vi "Script Editor Dialog.vi"(5 "VI Refnum":refnum<vi>, 7 "Name(\"\" to use uuid)":string="script_editor", 8 "Error in":errorcluster caption="Error in (no error)", 11 "Script":string="Data: Initialize\nInitialize Core Data\nEvents: Register\nUI: Initialize\nUI: Front Panel State >> Open") -> (0 "Error out":errorcluster, 3 "Script out":string)   [LabVIEW 2017]
uses:
  _Support/Priority Queue/Priority Queue.lvclass/Priority Queue.ctl
  AdvanceAPI/CSM - Keywords.vi
  _Support/Common/Trim Single line Text.vi
  AdvanceAPI/CSM - Check If Module Exists.vi
  Utility/Build Error Cluster.vi
  _Support/Process/CSMP-Sync Call.vi
  Utility/uuid.vi
  Utility/Trim Both Whitespace.vi
  _Support/CSMQ/_Obtain CSM Data Queue.vi
  _Support/Priority Queue/Release Priority Queue.vi
  _Support/CSMQ/_CSMObj-Message Check.vi
  _Support/CSMQ/_CSMObj-Enqueue Cross-Module Message.vi
  _Support/CSMQ/_CSMOFGV Get.vi
  _Support/Priority Queue/Obtain Priority Queue.vi
  _Support/Priority Queue/Enqueue Element.vi
  AdvanceAPI/CSM - Replace Substitution Marks in Messages.vi
  _Support/CSMQ/_CSMOFGV.vi
  _Support/Error/CSM No Target Error.vi
  _Support/Error/CSM Not Allowed Message.vi
  _Support/Message/global-TMO for Sync-Rep.vi
  _Support/Priority Queue/Priority Queue.lvclass
  Communicable State Machine.lvlib
panel:
  in  "Script List":i32(listbox)
  in  "Delete 3":bool
  in  "Delete 2":bool
  in  "Add Back":bool
  in  "Delete":bool
  in  "Add Front":bool
  in  "Replace":bool
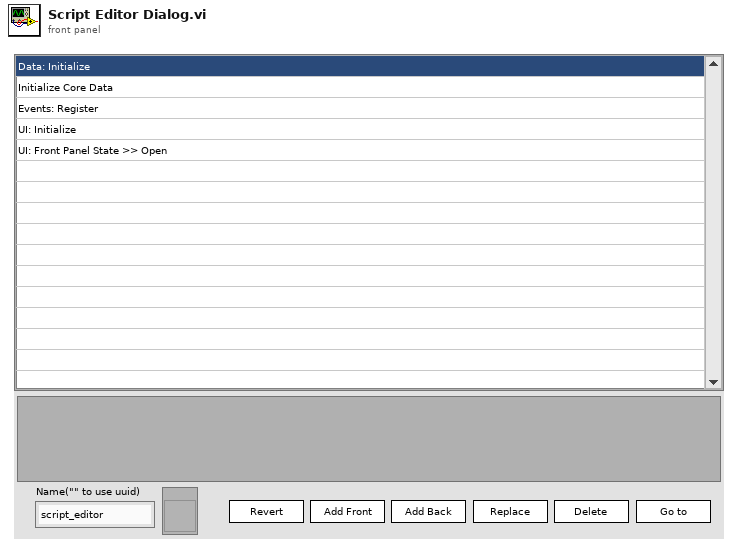
[diagram p1: front panel]
types:
  T1 = enum32{"Invalid", "Standard", "Closed", "Hidden", "Minimized", "Maximized"}
  T2 = enum32{"invalid app kind", "Development System", "Run Time System", "Student Edition", "Embedded LabVIEW", "Evaluation", "Custom"}
  T3 = typedef "Communicable State Machine.lvlib/_CSM_Response Source Message.ctl" = cluster{"‘State":string, "’Arguments":string, "’Error":errorcluster}
  T4 = cluster{"Current VI Reference":refnum<vi>, "Close Panel on Exit?":bool}
  T5 = cluster{"Core":cluster{"Current VI Reference":refnum<vi>, "Close Panel on Exit?":bool}, "Script":string}
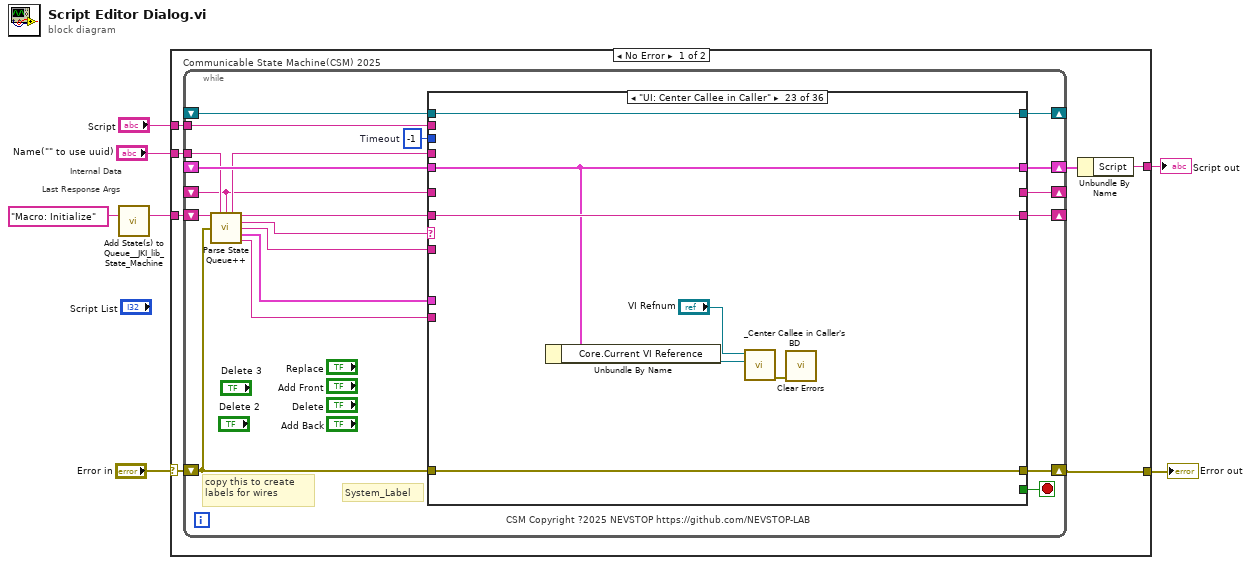
[diagram p0: block diagram]
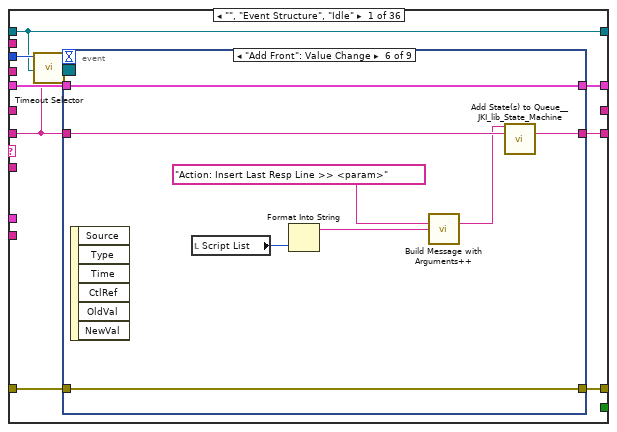
[diagram p2: hidden frame]
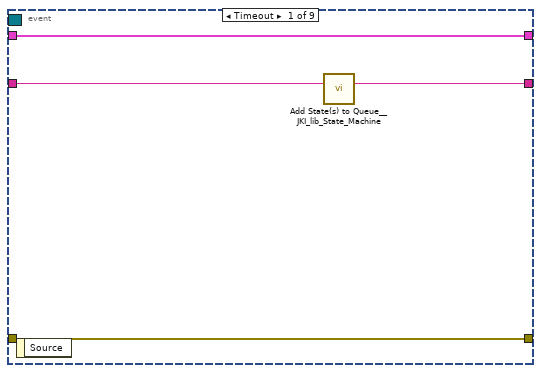
[diagram p3: hidden frame]
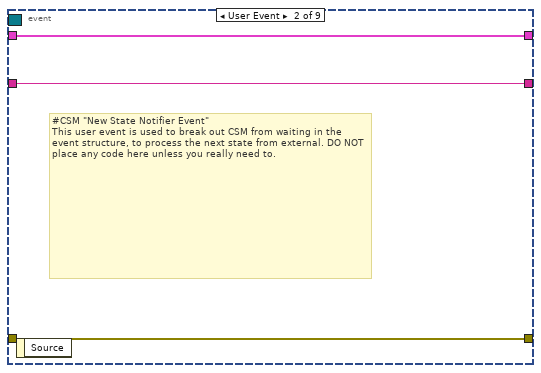
[diagram p4: hidden frame]
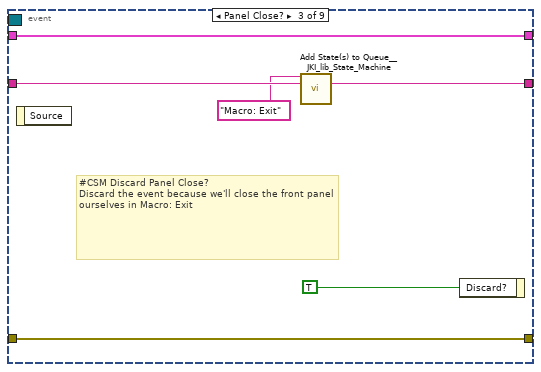
[diagram p5: hidden frame]
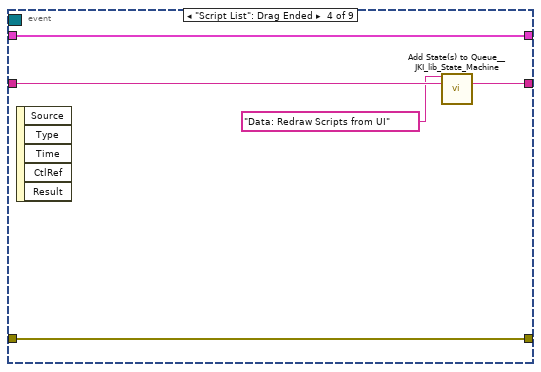
[diagram p6: hidden frame]
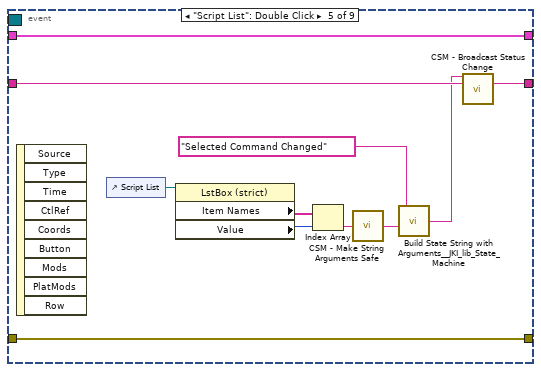
[diagram p7: hidden frame]
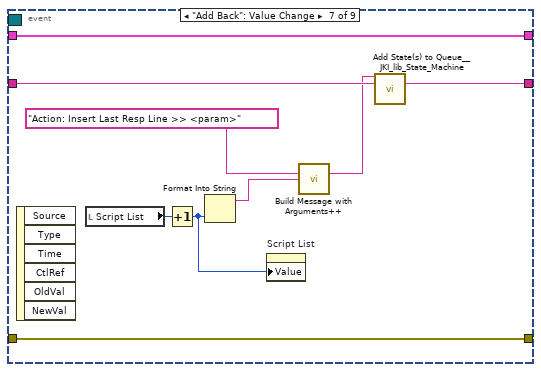
[diagram p8: hidden frame]
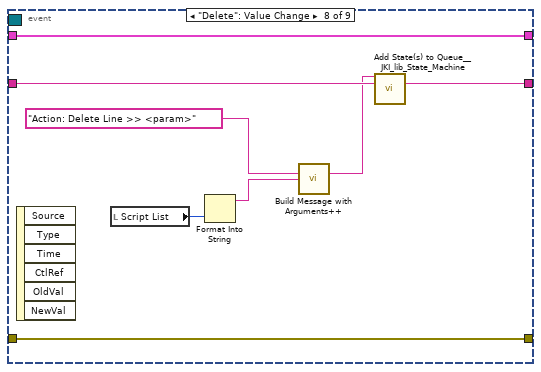
[diagram p9: hidden frame]
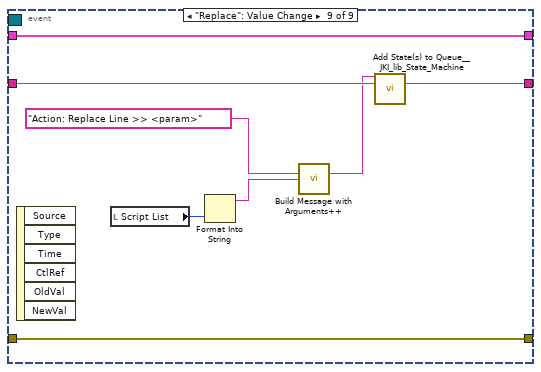
[diagram p10: hidden frame]
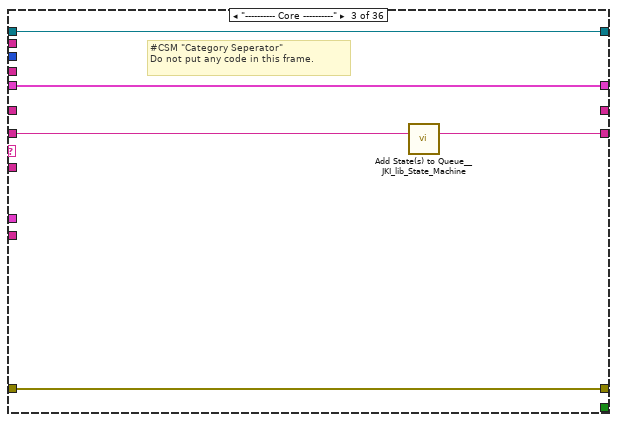
[diagram p12: hidden frame]
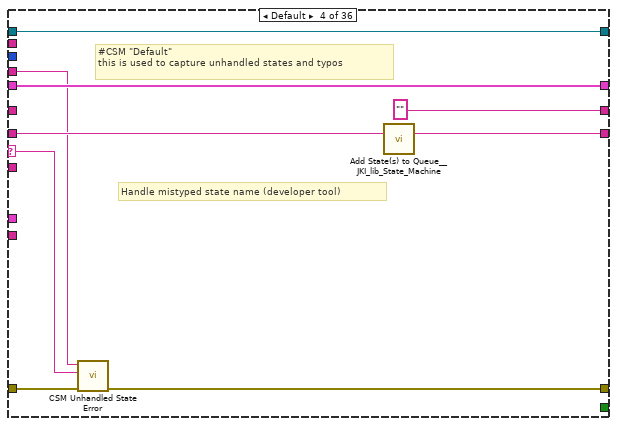
[diagram p13: hidden frame]
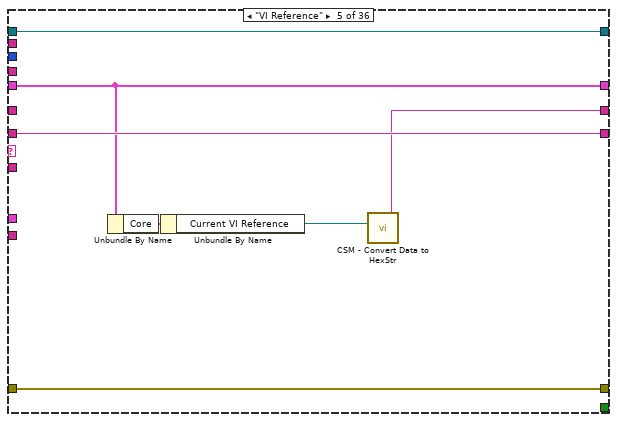
[diagram p14: hidden frame]
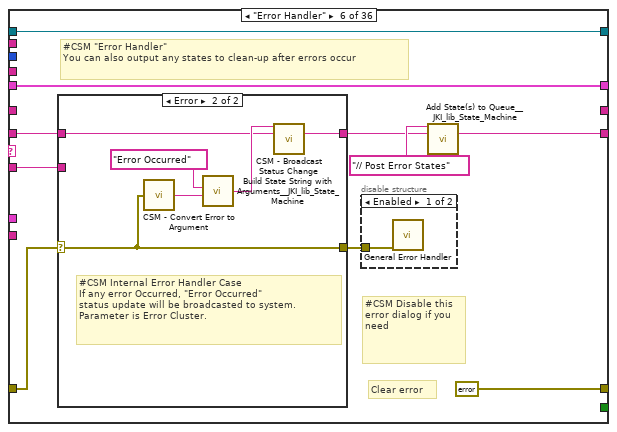
[diagram p15: hidden frame]
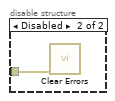
[diagram p16: hidden frame]
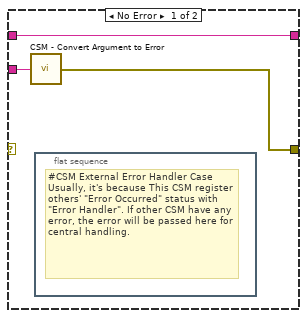
[diagram p17: hidden frame]
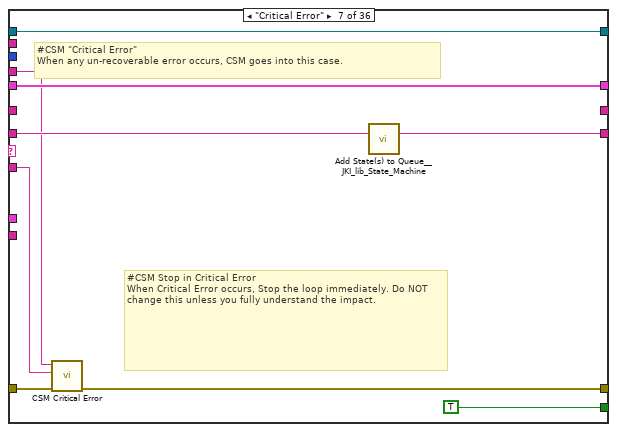
[diagram p18: hidden frame]
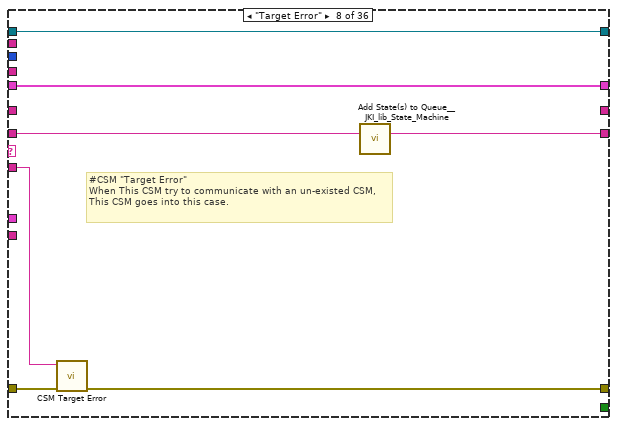
[diagram p19: hidden frame]
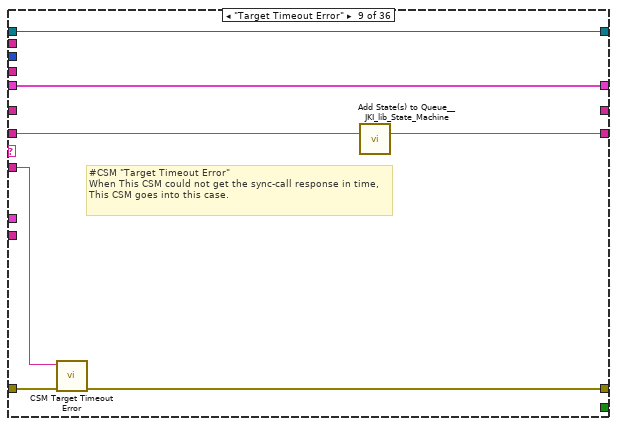
[diagram p20: hidden frame]
diagram:
  # "Last Response Args"
  # "Internal Data"
  n1 = call <vilib>:"Add State(s) to Queue__JKI_lib_State_Machine.vi"("State(s) in (\"\")"="Macro: Initialize" ("Init State(\"Macro: Initialize\")")) -> ("States Out"=w7:string)  [unwired: 14 in]
  n2 = case shown="No Error" "Error in" {
    selector: "Error in" -> [w11 w489]
    tunnel: w7 -> [w14 _]
    tunnel: "Name(\"\" to use uuid)" -> [w13 _]
    tunnel: [w12 w489] -> w4
    tunnel: [w9 w488] -> w2
    tunnel: "Script" -> [w8 w488]
    frame No Error {
      n3 = while "Communicable State Machine(CSM) 2025" {
        shift-right: [w29] -> w10
        shift-left: _ -> [w28]
        shift-right: [w32] -> w12
        shift-left: w11 -> [w26]
        shift-right: [w31] -> _
        shift-left: w14 -> [w33]
        tunnel: w13 -> [w22]
        shift-right: [w25] -> _
        shift-left: _ -> [w16]
        shift-right: [w24] -> _
        shift-left: _ -> [w23]
        tunnel: w8 -> [w15]
        stop <- w30 stop-if-true
        w27 = -1  # Timeout
        # "copy this to create labels for wires"
        # "System_Label"
        # "CSM Copyright ?2025 NEVSTOP https://github.com/NEVSTOP-LAB"
        n4 = call "Parse State Queue++.vi"("State Queue"=w33, "Name(\"\" to use uuid)"=w22, "Response Arguments"=w16, "Previous Error"=w26) -> ("Name Used"=w17:string, "Remaining States"=w34:string, "Current State"=w21:string, "Arguments"=w20:string, ">> Response Source Message >>"=w19:T3, ">> Source CSM >>"=w18:string)  [unwired: 6 in]
        n5 = case shown="\"UI: Center Callee in Caller\"" w21 {
          selector: w21 -> [_ _ _ w117 _ _ _ _ _ _ _ _ _ _ _ _ _ _ _ _ _ _ _ _ _ _ _ _ _ _ _ _ _ _ _ _]
          tunnel: w34 -> [w35 w108 w114 w122 w129 w135 w158 w164 w171 w180 w193 w208 w214 w219 w226 w233 w241 w246 w253 w257 w263 w270 w276 w279 w291 w307 w379 w401 w407 w421 w424 w427 w439 w457 w475 w487]
          tunnel: w20 -> [_ _ _ _ _ w134 w153 w163 w170 w179 _ _ _ _ _ _ _ _ _ _ _ _ _ _ w286 w301 _ _ _ _ _ w429 _ w453 w470 w482]
          tunnel: w28 -> [w42 w107 w111 w120 w128 w139 w159 w166 w173 w182 w192 w201 w212 w216 _ w232 w236 w243 w252 w256 w260 w266 w274 w283 w289 w303 w396 w398 w404 w418 w423 w433 w436 w455 w472 w484]
          tunnel: [w41 w109 w112 w115 w130 errorcluster {"status"=FALSE, "code"=0, "source"=""} ("error out") w154 w161 w168 w185 w194 w205 w211 w217 w223 w234 w237 w244 w247 w255 w261 w268 w277 w284 w287 w304 w378 w399 w405 w419 w425 w434 w437 w444 w473 w485] -> w32
          tunnel: w26 -> [w40 w109 w112 w123 w130 w136 w160 w162 w169 _ w194 w205 w211 w217 w223 w234 w238 w244 _ w258 w261 w268 w277 w284 w288 w305 _ w399 w405 w419 w425 w434 w437 _ w473 w485]
          tunnel: [w43 w108 w113 w121 w129 w131 w157 w167 w174 w181 w193 w207 w213 w218 w225 w233 w240 w245 w253 w257 w262 w269 w276 w280 w290 w306 w380 w400 w406 w420 w424 w428 w438 w456 w474 w486] -> w31
          tunnel: [_ _ _ _ _ _ TRUE _ _ _ _ _ TRUE _ _ _ _ _ _ _ _ _ _ _ _ _ _ _ _ _ _ _ _ _ _ _] -> w30
          tunnel: [w39 w107 w111 w120 w128 w139 w159 w166 w173 w183 w192 w206 w212 w216 w224 w228 w236 w243 w252 w256 w260 w266 w274 w283 w289 w303 w396 w398 w404 w418 w423 w431 w436 w455 w472 w484] -> w29
          tunnel: w27 -> [w38 _ _ _ _ _ _ _ _ _ _ _ _ _ _ _ _ _ _ _ _ _ _ _ _ _ _ _ _ _ _ _ _ _ _ _]
          tunnel: w18 -> [_ _ _ _ _ _ _ _ _ w177 _ _ _ _ _ _ _ _ _ _ _ _ _ _ _ _ _ _ _ _ _ _ _ _ _ _]
          tunnel: w19 -> [_ _ _ _ _ _ _ _ _ w184 _ _ _ _ _ _ _ _ _ _ _ _ _ _ _ _ _ _ _ _ _ _ _ _ _ _]
          tunnel: [_ _ _ "" w124 _ _ _ _ _ _ _ _ _ _ _ _ _ _ _ _ _ _ _ _ _ _ _ _ _ _ _ _ _ _ _] -> w25
          tunnel: [w37 w106 w110 w118 w127 w138 w155 w165 w172 w186 w191 w195 w209 w215 w221 w231 w235 w242 w251 w254 w259 w267 w275 w282 w285 w300 w395 w397 w402 w411 w422 w432 w435 w454 w471 w483] -> w24
          tunnel: w23 -> [w37 w106 w110 w118 w127 w138 w155 w165 w172 w186 w191 w195 w209 w215 w221 w231 w235 w242 _ w254 w259 w267 w275 w282 w285 w300 w395 w397 w402 w411 w422 w432 w435 w454 w471 w483]
          tunnel: w17 -> [_ _ _ w116 _ _ w152 _ _ _ _ _ _ _ _ _ _ _ w250 _ _ _ _ _ _ _ w384 _ _ w410 _ _ _ w443 w461 _]
          tunnel: w16 -> [_ _ _ _ _ _ _ _ _ _ _ _ _ _ _ _ _ _ _ _ _ _ _ _ _ _ _ _ _ _ _ _ _ _ _ _]
          tunnel: w15 -> [_ _ _ _ _ _ _ _ _ _ _ _ _ _ w220 _ _ _ _ _ _ _ _ _ _ _ _ _ _ _ _ _ _ _ _ _]
          frame "", "Event Structure", "Idle" {
            n6 = call "Timeout Selector.vi"("Remaining States"=w35, "Timeout Expected"=w38) -> ("Timeout"=w36:i32)  [unwired: 5 in]
            n7 = event shown="[5] \"Add Front\": Value Change" {
              selector: w37 -> [_ _ _ _ _ _ _ _ _]
              dyn-events: _ -> [_ _ _ _ _ _ _ _ _]
              timeout: w36 -> [_ _ _ _ _ _ _ _ _]
              tunnel: w35 -> [w47 w49 w56 w58 w69 w77 w86 w94 w102]
              tunnel: [w46 w49 w55 w59 w70 w78 w87 w95 w103] -> w43
              tunnel: w42 -> [w44 w50 w53 w60 w71 w79 w88 w96 w104]
              tunnel: [w45 w48 w54 w61 w72 w80 w89 w97 w105] -> w41
              tunnel: w40 -> [w45 w48 w54 w61 w72 w80 w89 w97 w105]
              tunnel: [w44 w50 w53 w60 w71 w79 w88 w96 w104] -> w39
              event Timeout {
                n8 = event-data() -> ()  [unwired: 1 in, 1 out]
                n9 = call <vilib>:"Add State(s) to Queue__JKI_lib_State_Machine.vi"("State(s) in (\"\")"=w47) -> ("States Out"=w46:string)  [unwired: 14 in]
              }
              event User Event {
                # "#CSM \"New State Notifier Event\"\nThis user event is used to break out CSM from waiting in the event structure, to process the next state from external. DO NOT place any code here unless you really need to."
                n10 = event-data() -> ()  [unwired: 1 in, 1 out]
              }
              event Panel Close? {
                # "#CSM Discard Panel Close?\nDiscard the event because we'll close the front panel ourselves in Macro: Exit"
                n11 = event-data() -> ()  [unwired: 1 in, 1 out]
                n12 = call <vilib>:"Add State(s) to Queue__JKI_lib_State_Machine.vi"("State(s) in Front (\"\")"="Macro: Exit", "State(s) in (\"\")"=w56) -> ("States Out"=w55:string)  [unwired: 13 in]
                n13 = event-data("Discard?"=TRUE) -> ()  [unwired: 1 in, 1 out]
              }
              event "Script List": Drag Ended {
                n14 = event-data() -> ()  [unwired: 1 in, 5 out]
                n15 = call <vilib>:"Add State(s) to Queue__JKI_lib_State_Machine.vi"("State(s) in Front (\"\")"="Data: Redraw Scripts from UI" ("State(s) in Front (\"\")"), "State(s) in (\"\")"=w58) -> ("States Out"=w59:string)  [unwired: 13 in]
              }
              event "Script List": Double Click {
                n16 = event-data() -> ()  [unwired: 1 in, 9 out]
                n17 = control-ref of="Script List"() -> (w65:refnum<vi>)
                n18 = property class="LstBox (strict)"(reference=w65) -> ("Item Names"=w68:string[], "Value"=w67:i32)  [unwired: 1 in, 2 out]
                n19 = Index Array(array=w68, index=w67) -> (element=w66:string)
                n20 = call "CSM - Make String Arguments Safe.vi"("Argurment String"=w66) -> ("Safe Argurment String"=w64:string)  [unwired: 8 in]
                n21 = call <vilib>:"Build State String with Arguments__JKI_lib_State_Machine.vi"("Arguments (\"\")"=w64, "State"="Selected Command Changed") -> ("State with Arguments"=w62:string)  [unwired: 4 in]
                n22 = call "CSM - Broadcast Status Change.vi"("Status with Arguments"=w62, "State Queue"=w69) -> ("Remaining States"=w70:string)  [unwired: 13 in]
              }
              event "Add Front": Value Change {
                n23 = event-data() -> ()  [unwired: 1 in, 6 out]
                n24 = local read "Script List"() -> (w74:i32)
                n25 = Format Into String(w74) -> (resulting string=w73:string)  [unwired: 3 in, 1 out]
                n26 = call-poly "Build Message with Arguments++.vi"("States with Replace Token"="Action: Insert Last Resp Line >> <param>" ("State(s) in Front (\"\")"), "<param>"=w73) -> ("States"=w75:string)  [unwired: 13 in]
                n27 = call <vilib>:"Add State(s) to Queue__JKI_lib_State_Machine.vi"("State(s) in Front (\"\")"=w75, "State(s) in (\"\")"=w77) -> ("States Out"=w78:string)  [unwired: 13 in]
              }
              event "Add Back": Value Change {
                n28 = event-data() -> ()  [unwired: 1 in, 6 out]
                n29 = local read "Script List"() -> (w83:i32)
                n30 = Increment(x=w83) -> (x+1=w81:i32)
                n31 = Format Into String(w81) -> (resulting string=w82:string)  [unwired: 3 in, 1 out]
                n32 = property on="Script List" class="LstBox (strict)"("Value"=w81) -> ()  [unwired: 2 in, 2 out]
                n33 = call-poly "Build Message with Arguments++.vi"("States with Replace Token"="Action: Insert Last Resp Line >> <param>" ("State(s) in Front (\"\")"), "<param>"=w82) -> ("States"=w84:string)  [unwired: 13 in]
                n34 = call <vilib>:"Add State(s) to Queue__JKI_lib_State_Machine.vi"("State(s) in Front (\"\")"=w84, "State(s) in (\"\")"=w86) -> ("States Out"=w87:string)  [unwired: 13 in]
              }
              event "Delete": Value Change {
                n35 = event-data() -> ()  [unwired: 1 in, 6 out]
                n36 = local read "Script List"() -> (w91:i32)
                n37 = Format Into String(w91) -> (resulting string=w90:string)  [unwired: 3 in, 1 out]
                n38 = call-poly "Build Message with Arguments++.vi"("States with Replace Token"="Action: Delete Line >> <param>" ("State(s) in Front (\"\")"), "<param>"=w90) -> ("States"=w92:string)  [unwired: 13 in]
                n39 = call <vilib>:"Add State(s) to Queue__JKI_lib_State_Machine.vi"("State(s) in Front (\"\")"=w92, "State(s) in (\"\")"=w94) -> ("States Out"=w95:string)  [unwired: 13 in]
              }
              event "Replace": Value Change {
                n40 = event-data() -> ()  [unwired: 1 in, 6 out]
                n41 = local read "Script List"() -> (w99:i32)
                n42 = Format Into String(w99) -> (resulting string=w98:string)  [unwired: 3 in, 1 out]
                n43 = call-poly "Build Message with Arguments++.vi"("States with Replace Token"="Action: Replace Line >> <param>" ("State(s) in Front (\"\")"), "<param>"=w98) -> ("States"=w100:string)  [unwired: 13 in]
                n44 = call <vilib>:"Add State(s) to Queue__JKI_lib_State_Machine.vi"("State(s) in Front (\"\")"=w100, "State(s) in (\"\")"=w102) -> ("States Out"=w103:string)  [unwired: 13 in]
              }
            }
          }
          frame "CSM Documentation" {
            # "#CSM README FIRST\n\nCommunicable State Machine(CSM) is a LabVIEW application framework that builds upon JKI State Machine(JKISM). It follows the pattern of JKISM and extends the keywords to describe message communication between modules, including concepts such as Sync-Message, Async-Message, Subscription/Unsubscription of status - essential elements for creating reusable code modules. For more information, please visit the CSM wiki: https://nevstop-lab.github.io/CSM-Wiki/\n\nFor instructions on JKI State Machine, visit: http://jki.net/state-machine/\nFor information about CSM, visit: https://github.com/NEVSTOP-LAB"
            # "#CSM \"Documentation\"\nCase for holding CSM Documenation"
          }
          frame "---------- Core ----------" {
            # "#CSM \"Category Seperator\"\nDo not put any code in this frame."
            n45 = call <vilib>:"Add State(s) to Queue__JKI_lib_State_Machine.vi"("State(s) in (\"\")"=w114) -> ("States Out"=w113:string)  [unwired: 14 in]
          }
          frame Default {
            # "#CSM \"Default\"\nthis is used to capture unhandled states and typos"
            # "Handle mistyped state name (developer tool)"
            n46 = call "CSM Unhandled State Error.vi"("error in (no error)"=w123, "Current State"=w117, "CSM Name"=w116) -> ("error out"=w115:errorcluster)  [unwired: 8 in]
            n47 = call <vilib>:"Add State(s) to Queue__JKI_lib_State_Machine.vi"("State(s) in (\"\")"=w122) -> ("States Out"=w121:string)  [unwired: 14 in]
          }
          frame "VI Reference" {
            n48 = Unbundle By Name(w128) -> ("Core"=w126:T4)
            n49 = Unbundle By Name(w126) -> ("Current VI Reference"=w125:refnum<vi>)
            n50 = call "CSM - Convert Data to HexStr.vi"("Variant"=w125) -> ("HEX String (0-9,A-F)"=w124:string)  [unwired: 8 in]
          }
          frame "Error Handler" {
            # "#CSM Disable this error dialog if you need"
            # "#CSM \"Error Handler\"\nYou can also output any states to clean-up after errors occur"
            # "Clear error"
            n51 = case shown="Error" w136 {
              selector: w136 -> [_ w146]
              tunnel: [w145 w148] -> w132
              tunnel: w135 -> [w145 w147]
              tunnel: w134 -> [w144 _]
              tunnel: [w143 w146] -> w137
              frame No Error {
                n52 = call "CSM - Convert Argument to Error.vi"("Argument"=w144) -> ("error"=w143:errorcluster)  [unwired: 4 in]
                n53 = flat-sequence {
                  frame #0 {
                    # "#CSM External Error Handler Case\nUsually, it's because This CSM register others' \"Error Occurred\" status with \"Error Handler\". If other CSM have any error, the error will be passed here for central handling."
                  }
                }
              }
              frame Error {
                # "#CSM Internal Error Handler Case \nIf any error Occurred, \"Error Occurred\" \nstatus update will be broadcasted to system.\nParameter is Error Cluster."
                n54 = call "CSM - Convert Error to Argument.vi"("error"=w146) -> ("Argument"=w150:string)  [unwired: 4 in]
                n55 = call <vilib>:"Build State String with Arguments__JKI_lib_State_Machine.vi"("Arguments (\"\")"=w150, "State"="Error Occurred" ("Status with Arguments")) -> ("State with Arguments"=w149:string)  [unwired: 4 in]
                n56 = call "CSM - Broadcast Status Change.vi"("Status with Arguments"=w149, "State Queue"=w147) -> ("Remaining States"=w148:string)  [unwired: 13 in]
              }
            }
            n57 = disable-structure shown="Enabled" {
              disable-tunnel: w137 -> [w141 w142]
              frame Enabled {
                n58 = call <vilib>:"General Error Handler.vi"("error in (no error)"=w141) -> ()  [unwired: 10 in, 5 out]
              }
              frame Disabled {
                n59 = call <vilib>:"Clear Errors.vi"("error in (no error)"=w142) -> ()  [unwired: 5 in, 2 out]
              }
            }
            n60 = call <vilib>:"Add State(s) to Queue__JKI_lib_State_Machine.vi"("State(s) in Front (\"\")"="// Post Error States", "State(s) in (\"\")"=w132) -> ("States Out"=w131:string)  [unwired: 13 in]
          }
          frame "Critical Error" {
            # "#CSM Stop in Critical Error\nWhen Critical Error occurs, Stop the loop immediately. Do NOT change this unless you fully understand the impact."
            # "#CSM \"Critical Error\"\nWhen any un-recoverable error occurs, CSM goes into this case."
            n61 = call "CSM Critical Error.vi"("error in (no error)"=w160, "Arugments(as Reason)"=w153, "CSM Name"=w152) -> ("error out"=w154:errorcluster)  [unwired: 8 in]
            n62 = call <vilib>:"Add State(s) to Queue__JKI_lib_State_Machine.vi"("State(s) in (\"\")"=w158) -> ("States Out"=w157:string)  [unwired: 14 in]
          }
          frame "Target Error" {
            # "#CSM \"Target Error\"\nWhen This CSM try to communicate with an un-existed CSM, This CSM goes into this case."
            n63 = call "CSM Target Error.vi"("error in (no error)"=w162, "Arguments(as CSM Name)"=w163) -> ("error out"=w161:errorcluster)  [unwired: 9 in]
            n64 = call <vilib>:"Add State(s) to Queue__JKI_lib_State_Machine.vi"("State(s) in (\"\")"=w164) -> ("States Out"=w167:string)  [unwired: 14 in]
          }
          frame "Target Timeout Error" {
            # "#CSM \"Target Timeout Error\"\nWhen This CSM could not get the sync-call response in time, This CSM goes into this case."
            n65 = call "CSM Target Timeout Error.vi"("error in (no error)"=w169, "Arguments(as CSM Name)"=w170) -> ("error out"=w168:errorcluster)  [unwired: 9 in]
            n66 = call <vilib>:"Add State(s) to Queue__JKI_lib_State_Machine.vi"("State(s) in (\"\")"=w171) -> ("States Out"=w174:string)  [unwired: 14 in]
          }
          frame "Async Response", "Response" {
            n67 = Unbundle(w184) -> ("‘State"=w178:string, "’Arguments"=w176:string, "’Error"=w175:errorcluster)
            n68 = case shown="Default" w178 {
              tunnel: [w190] -> w185
              tunnel: w175 -> [w190]
              tunnel: [w189] -> w183
              tunnel: w182 -> [w189]
              tunnel: [w187] -> w181
              tunnel: w180 -> [w188]
              tunnel: w179 -> [_]
              tunnel: w177 -> [_]
              tunnel: w176 -> [_]
              frame Default {
                # "#CSM Response Comments\nAfter Message is executed, CSM goes to this state for receive the response.\n    For Async Message(->), \"Async Response\" is used. This CSM will goes to \"Async Message Posted\" immediately and receive the \"Async Response\" after the callee finishes the message.\n    For Sync Message(@),  This CSM will wait until the message is done and immediately goes to \"Response\""
                # "#CSM \"Async Response\"\nHandle Async-call Response (\"Async Response\" for ->)"
                # "#CSM \"Response\"\nHandle Sync-call Response (\"Response\" for -@)"
                n69 = call <vilib>:"Add State(s) to Queue__JKI_lib_State_Machine.vi"("State(s) in (\"\")"=w188) -> ("States Out"=w187:string)  [unwired: 14 in]
              }
            }
          }
          frame "Async Message Posted" {
            # "#CSM \"Async Message Posted\"\nAfter Async Message is posted (-> or ->| ), CSM goes to this state for post-action.\nYou can use Argument - State to tell which Async Message is called."
          }
          frame "Initialize Core Data" {
            # "#CSM \"Initialize Core Data\"\nThis is used to determine panel behavior on exit"
            # "originally closed?"
            # "exe?"
            # "If panel starts closed or is an EXE, then close it when we exit"
            n70 = property class="VI"() -> ("FP.State"=w198:T1)  [unwired: 2 in, 2 out]
            n71 = property class="App"() -> ("App.Kind"=w204:T2)  [unwired: 2 in, 2 out]
            n72 = control-ref of="Current VI Reference"() -> (w199:refnum<vi>)
            n73 = Equal?(x=w198, y=T1."Closed" ("Front Panel Window:State")) -> (x = y?=w196:bool)
            n74 = Equal?(x=w204, y=T2."Run Time System" ("Application:Kind")) -> (x = y?=w202:bool)
            n75 = Or(x=w196, y=w202) -> (x .or. y?=w200:bool)
            n76 = Bundle By Name(cluster=w201, "Core.Current VI Reference"=w199, "Core.Close Panel on Exit?"=w200) -> (w206:T5)
            n77 = call <vilib>:"Add State(s) to Queue__JKI_lib_State_Machine.vi"("State(s) in (\"\")"=w208) -> ("States Out"=w207:string)  [unwired: 14 in]
          }
          frame "Exit" {
            # "#CSM \"Exit\"\nCase for exiting the loop. No errors that occur here will be handled."
            n78 = call <vilib>:"Add State(s) to Queue__JKI_lib_State_Machine.vi"("State(s) in (\"\")"=w214) -> ("States Out"=w213:string)  [unwired: 14 in]
          }
          frame "---------- Data ----------" {
            # "#CSM \"Category Seperator\"\nDo not put any code in this frame."
            n79 = call <vilib>:"Add State(s) to Queue__JKI_lib_State_Machine.vi"("State(s) in (\"\")"=w219) -> ("States Out"=w218:string)  [unwired: 14 in]
          }
          frame "Data: Initialize" {
            w222 = T4 {"Current VI Reference"=refnum, "Close Panel on Exit?"=FALSE}  # Core
            n80 = Bundle("Core"=w222, "Script"=w220) -> (w224:T5)  [unwired: 1 in]
            n81 = call <vilib>:"Add State(s) to Queue__JKI_lib_State_Machine.vi"("State(s) in (\"\")"=w226) -> ("States Out"=w225:string)  [unwired: 14 in]
          }
          frame "Data: Redraw Scripts from UI" {
            n82 = control-ref of="Script List"() -> (w230:refnum<vi>)
            n83 = property class="LstBox (strict)"(reference=w230) -> ("Item Names"=w229:string[])  [unwired: 1 in, 2 out]
            n84 = call "CSM - Compact Multiple States.vi"("Multiple States"=w229) -> ("States"=w227:string)  [unwired: 9 in]
            n85 = Bundle By Name(cluster=w232, "Script"=w227) -> (w228:T5)
          }
          frame "Data: Cleanup" {
            # "Cleanup any data and references, here.\n(this is called automatically, by the Macro: Exit)"
            n86 = Unbundle By Name(w236) -> ("Core.Current VI Reference"=w239:refnum<vi>)
            n87 = Close Reference(reference=w239, error in (no error)=w238) -> (error out=w237:errorcluster)
            n88 = call <vilib>:"Add State(s) to Queue__JKI_lib_State_Machine.vi"("State(s) in (\"\")"=w241) -> ("States Out"=w240:string)  [unwired: 14 in]
          }
          frame "---------- Events ----------" {
            # "#CSM \"Category Seperator\"\nDo not put any code in this frame."
            n89 = call <vilib>:"Add State(s) to Queue__JKI_lib_State_Machine.vi"("State(s) in (\"\")"=w246) -> ("States Out"=w245:string)  [unwired: 14 in]
          }
          frame "Events: Register" {
            # "#CSM \"Events: Register\"\nRegister user event. New Message Event is registered to break CSM waiting in event structure by default."
            # "#CSM Register New Message Event\nRegister message event to break Waiting in Event structure."
            n90 = call "CSM - Get New State Notifier Event.vi"("Name(\"\" to use uuid) in"=w250) -> ("Error out"=w248:errorcluster, "New State Notifier Event"=w249:refnum<user-event>)  [unwired: 9 in]
            n91 = register-events(error in=w248, w249) -> (reference out=w251:refnum<event-registration>, error out=w247:errorcluster)  [unwired: 1 in]
          }
          frame "Events: Unregister" {
            # "#CSM \"Events: Unregister\"\nUnregister user event."
            n92 = Unregister For Events(event registration refnum=w254, error in=w258) -> (error out=w255:errorcluster)
          }
          frame "---------- UI ----------" {
            # "#CSM \"Category Seperator\"\nDo not put any code in this frame."
            n93 = call <vilib>:"Add State(s) to Queue__JKI_lib_State_Machine.vi"("State(s) in (\"\")"=w263) -> ("States Out"=w262:string)  [unwired: 14 in]
          }
          frame "UI: Initialize" {
            # "#CSM \"UI: Initialize\"\nInitialize the User Interface, here.\n(this is called automatically, by the Macro: Init)"
            n94 = Unbundle By Name(w266) -> ("Script"=w265:string)
            n95 = call "CSM - Break Down Multiple States String.vi"("States"=w265) -> ("Multiple States"=w264:string[])  [unwired: 10 in]
            n96 = property on="Script List" class="LstBox (strict)"("Item Names"=w264) -> ()  [unwired: 2 in, 2 out]
            n97 = call <vilib>:"Add State(s) to Queue__JKI_lib_State_Machine.vi"("State(s) in (\"\")"=w270) -> ("States Out"=w269:string)  [unwired: 14 in]
          }
          frame "UI: Center Callee in Caller" {
            n98 = Unbundle By Name(w274) -> ("Core.Current VI Reference"=w271:refnum<vi>)
            n99 = call "_Center Callee in Caller's BD.vi"("Callee VI Refnum (Caller)"=w271, "Caller VI Refnum (Callee's Caller)"="VI Refnum") -> ("Error Out"=w273:errorcluster)  [unwired: 9 in]
            n100 = call <vilib>:"Clear Errors.vi"("error in (no error)"=w273) -> ()  [unwired: 5 in, 2 out]
          }
          frame "UI: Refresh Inputs" {
            n101 = call <vilib>:"Build State String with Arguments__JKI_lib_State_Machine.vi"("State"="") -> ("State with Arguments"=w278:string)  [unwired: 5 in]
            n102 = call <vilib>:"Add State(s) to Queue__JKI_lib_State_Machine.vi"("State(s) in Front (\"\")"=w278, "State(s) in (\"\")"=w279) -> ("States Out"=w280:string)  [unwired: 13 in]
          }
          frame "UI: Cursor Set" {
            # "#CSM \"UI: Cursor Set\"\nSet and Unset Cursor Busy.\n(Usage: \"UI: Cursor Set >> Busy|Idle\")"
            # "Argument"
            n103 = disable-structure shown="Default" {
              disable-tunnel: w288 -> [w294 w299]
              disable-tunnel: [w293 w299] -> w287
              disable-tunnel: w286 -> [w292 _]
              frame condition #0 (active) {
                n104 = case shown="\"Idle\", Default" w292 {
                  tunnel: w294 -> [w296 w298]
                  tunnel: [w295 w297] -> w293
                  frame "Idle", Default {
                    n105 = call <vilib>:"Unset Busy.vi"("error in (no error)"=w296) -> ("error out"=w295:errorcluster)  [unwired: 10 in]
                  }
                  frame "Busy" {
                    n106 = call <vilib>:"Set Busy.vi"("error in (no error)"=w298) -> ("error out"=w297:errorcluster)  [unwired: 9 in, 1 out]
                  }
                }
              }
              frame condition #1 {
              }
            }
            n107 = call <vilib>:"Add State(s) to Queue__JKI_lib_State_Machine.vi"("State(s) in (\"\")"=w291) -> ("States Out"=w290:string)  [unwired: 14 in]
          }
          frame "UI: Front Panel State" {
            # "#CSM \"UI: Front Panel State\"\nSet Front Panel Open or Closed\n(Usage: \"UI: Front Panel State >> Open|Close\")"
            # "Argument"
            n108 = Unbundle By Name(w303) -> ("Core.Current VI Reference"=w302:refnum<vi>)
            n109 = call <vilib>:"Add State(s) to Queue__JKI_lib_State_Machine.vi"("State(s) in (\"\")"=w307) -> ("States Out"=w306:string)  [unwired: 14 in]
            n110 = case shown="\"Close\", \"Closed\"" w301 {
              tunnel: w305 -> [w313 w328 w339 w352 w365]
              tunnel: [w315 w329 w341 w354 w367] -> w304
              tunnel: w302 -> [w314 w326 w340 w353 w366]
              frame "Open", "Standard", Default {
                w308 = T1."Standard" ("State")
                n111 = property class="VI"(reference=w314, error in=w313) -> (reference out=w311:refnum<vi>, error out=w312:errorcluster, "FP.State"=w310:T1)
                n112 = Not Equal?(x=w310, y=w308) -> (x != y?=w309:bool)
                n113 = case shown="True" w309 {
                  tunnel: [w319 w321] -> w315
                  tunnel: w312 -> [w318 w321]
                  tunnel: w311 -> [w317 _]
                  tunnel: w308 -> [w316 _]
                  frame True {
                    n114 = invoke class="VI" method="FP.Open"(reference=w317, error in=w318, "Activate"=TRUE, "State"=w316) -> (error out=w319:errorcluster)  [unwired: 1 in, 4 out]
                  }
                  frame False {
                  }
                }
              }
              frame "Close", "Closed" {
                n115 = property class="VI"(reference=w326, error in=w328) -> (reference out=w325:refnum<vi>, error out=w327:errorcluster, "FP.State"=w323:T1)
                n116 = Not Equal?(x=w323, y=T1."Closed" ("Front Panel Window:State")) -> (x != y?=w322:bool)
                n117 = case shown="False" w322 {
                  tunnel: [w330 w333] -> w329
                  tunnel: w327 -> [w330 w332]
                  tunnel: w325 -> [_ w331]
                  frame False {
                  }
                  frame True {
                    n118 = invoke class="VI" method="FP.Close"(reference=w331, error in=w332) -> (error out=w333:errorcluster)  [unwired: 1 in, 2 out]
                  }
                }
              }
              frame "Hidden", "Hide" {
                w334 = T1."Hidden" ("State")
                n119 = property class="VI"(reference=w340, error in=w339) -> (reference out=w337:refnum<vi>, error out=w338:errorcluster, "FP.State"=w336:T1)
                n120 = Not Equal?(x=w336, y=w334) -> (x != y?=w335:bool)
                n121 = case shown="True" w335 {
                  tunnel: [w345 w346] -> w341
                  tunnel: w338 -> [w344 w346]
                  tunnel: w337 -> [w343 _]
                  tunnel: w334 -> [w342 _]
                  frame True {
                    n122 = invoke class="VI" method="FP.Open"(reference=w343, error in=w344, "State"=w342) -> (error out=w345:errorcluster)  [unwired: 2 in, 4 out]
                  }
                  frame False {
                  }
                }
              }
              frame "Minimize", "Minimized" {
                w347 = T1."Minimized" ("State")
                n123 = property class="VI"(reference=w353, error in=w352) -> (reference out=w350:refnum<vi>, error out=w351:errorcluster, "FP.State"=w349:T1)
                n124 = Not Equal?(x=w349, y=w347) -> (x != y?=w348:bool)
                n125 = case shown="True" w348 {
                  tunnel: [w358 w359] -> w354
                  tunnel: w351 -> [w357 w359]
                  tunnel: w350 -> [w356 _]
                  tunnel: w347 -> [w355 _]
                  frame True {
                    n126 = invoke class="VI" method="FP.Open"(reference=w356, error in=w357, "State"=w355) -> (error out=w358:errorcluster)  [unwired: 2 in, 4 out]
                  }
                  frame False {
                  }
                }
              }
              frame "Maximize", "Maximized" {
                w360 = T1."Maximized" ("State")
                n127 = property class="VI"(reference=w366, error in=w365) -> (reference out=w363:refnum<vi>, error out=w364:errorcluster, "FP.State"=w362:T1)
                n128 = Not Equal?(x=w362, y=w360) -> (x != y?=w361:bool)
                n129 = case shown="True" w361 {
                  tunnel: [w371 w372] -> w367
                  tunnel: w364 -> [w370 w372]
                  tunnel: w363 -> [w369 _]
                  tunnel: w360 -> [w368 _]
                  frame True {
                    n130 = invoke class="VI" method="FP.Open"(reference=w369, error in=w370, "State"=w368) -> (error out=w371:errorcluster)  [unwired: 2 in, 4 out]
                  }
                  frame False {
                  }
                }
              }
            }
          }
          frame "UI: Insert Command Editor Dialog" {
            n131 = vi-ref "Command Editor Dialog.vi"() -> (w385:refnum<vi>)
            n132 = property class="VI (strict)"(reference=w385) -> (reference out=w390:refnum<vi>, error out=w388:errorcluster, "Path"=w387:path)  [unwired: 1 in]
            n133 = Open VI Reference(type specifier VI Refnum (for type only)=w390, vi path=w387, options=128, error in (no error)=w388) -> (vi reference=w389:refnum<vi>, error out=w386:errorcluster)  [unwired: 2 in]
            n134 = call "Concatenate Submodule Name.vi"("name"="CmdEditor", "CSM Name"=w384) -> ("submodule name"=w373:string)  [unwired: 9 in]
            n135 = call-by-ref "Start Asynchronous Call"(reference=w389, error in=w386, "Name(\"\" to use uuid)"=w373, "Command"="") -> (reference out=w393:refnum<vi>, error out=w392:errorcluster)  [unwired: 8 in, 2 out]
            n136 = Close Reference(reference=w393, error in (no error)=w392) -> (error out=w383:errorcluster)
            n137 = call "CSM - Wait for Module to Be Alive.vi"("CSM Name"=w373, "error in (no error)"=w383) -> ("CSM Name(dup)"=w381:string, "error out"=w382:errorcluster)  [unwired: 11 in, 1 out]
            n138 = call "CSM - Module VI Reference.vi"("error in (no error)"=w382, "CSM Name"=w381) -> ("CSM Module VIRef"=w376:refnum<vi>)  [unwired: 8 in, 1 out]
            n139 = invoke on="Sub Panel" class="SubPnl" method="Insert VI"("VI Ref"=w376) -> (error out=w378:errorcluster)  [unwired: 3 in, 3 out]
            n140 = call-poly "Build Message with Arguments++.vi"("States with Replace Token"="Selected Command changed@* >> API: Set Command@<target>-><register>" ("State(s) in Front (\"\")"), "<target>"=w373) -> ("States"=w375:string)  [unwired: 13 in]
            n141 = call <vilib>:"Add State(s) to Queue__JKI_lib_State_Machine.vi"("State(s) in Front (\"\")"=w375, "State(s) in (\"\")"=w379) -> ("States Out"=w380:string)  [unwired: 13 in]
          }
          frame "---------- Macro ----------" {
            # "#CSM \"Category Seperator\"\nDo not put any code in this frame."
            n142 = call <vilib>:"Add State(s) to Queue__JKI_lib_State_Machine.vi"("State(s) in (\"\")"=w401) -> ("States Out"=w400:string)  [unwired: 14 in]
          }
          frame "Macro: Initialize" {
            w403 = "Data: Initialize\nInitialize Core Data\nEvents: Register\nUI: Initialize\nUI: Front Panel State >> Open\nUI: Center Callee in Caller\nUI: Insert Command Editor Dialog"  # Data: Initialize Initialize Core Data Events: Register UI: Initialize UI: Front Panel State >> Open UI: Center Callee in Caller UI: Insert Command Editor Dialog
            # "#CSM \"Macro: Initialize\"\nInitialization Macro (This is called once, when the VI starts)"
            n143 = call <vilib>:"Add State(s) to Queue__JKI_lib_State_Machine.vi"("State(s) in Front (\"\")"=w403, "State(s) in (\"\")"=w407) -> ("States Out"=w406:string)  [unwired: 13 in]
          }
          frame "Macro: Exit" {
            # "#CSM \"Macro: Exit\"\nExit Macro (This is called once, when the VI exits)"
            n144 = Unbundle By Name(w418) -> ("Core.Close Panel on Exit?"=w417:bool)
            n145 = call "CSM - List Submodules.vi"("CSM Name"=w410) -> ("submodules"=w409:string[])  [unwired: 8 in, 2 out]
            n146 = call "CSM - Build Exit Messages of CSMs.vi"("CSMs"=w409) -> ("States"=w408:string)  [unwired: 14 in]
            n147 = Select(t="UI: Front Panel State >> Close", s=w417, f="") -> (s? t:f=w414:string)
            n148 = call <vilib>:"Add State(s) to Queue__JKI_lib_State_Machine.vi"("State(s) in Front (\"\")"=w408, "State(s) in (\"\")"=w414, "State(s) at Back (\"\")"="Data: Cleanup\nEvents: Unregister\nExit") -> ("States Out"=w412:string)  [unwired: 12 in]
            n149 = call <vilib>:"Add State(s) to Queue__JKI_lib_State_Machine.vi"("State(s) in Front (\"\")"=w412, "State(s) in (\"\")"=w421) -> ("States Out"=w420:string)  [unwired: 13 in]
          }
          frame "---------- API ----------" {
            # "#CSM \"Category Seperator\"\nDo not put any code in this frame."
          }
          frame "API: Set Script" {
            # "#CSM API Example\nCopy/Rename this case for your own API"
            n150 = call "CSM - Revert Arguments-Safe String.vi"("Safe Argurment String"=w429) -> ("Origin Argurment String"=w430:string)  [unwired: 8 in]
            n151 = Bundle By Name(cluster=w433, "Script"=w430) -> (w431:T5)
            n152 = call <vilib>:"Add State(s) to Queue__JKI_lib_State_Machine.vi"("State(s) in (\"\")"=w427, "State(s) at Back (\"\")"="UI: Refresh Inputs" ("State(s) in Front (\"\")")) -> ("States Out"=w428:string)  [unwired: 13 in]
          }
          frame "---------- Action ----------" {
            # "#CSM \"Category Seperator\"\nDo not put any code in this frame."
            n153 = call <vilib>:"Add State(s) to Queue__JKI_lib_State_Machine.vi"("State(s) in (\"\")"=w439) -> ("States Out"=w438:string)  [unwired: 14 in]
          }
          frame "Action: Insert Last Resp Line" {
            n154 = Decimal String To Number(string=w453) -> (number=w450:i32)  [unwired: 2 in, 1 out]
            n155 = control-ref of="Script List"() -> (w452:refnum<vi>)
            n156 = call "Concatenate Submodule Name.vi"("name"="CmdEditor", "CSM Name"=w443) -> ("submodule name"=w441:string)  [unwired: 9 in]
            n157 = property class="LstBox (strict)"(reference=w452) -> (reference out=w448:refnum<vi>, "Item Names"=w451:string[])  [unwired: 1 in, 1 out]
            n158 = call "CSM - Send Message and Wait for Reply.vi"("Current Module(\"\" to generate a ID)"=w443, "Target Module"=w441, "State"="API: Get Command") -> ("error out"=w444:errorcluster, "Response"=w446:string)  [unwired: 6 in, 1 out]
            n159 = call "CSM - Revert Arguments-Safe String.vi"("Safe Argurment String"=w446) -> ("Origin Argurment String"=w445:string)  [unwired: 8 in]
            n160 = Insert Into Array(array=w451, index=w450, new element=w445) -> (w449:string[])
            n161 = property class="LstBox (strict)"(reference=w448, "Item Names"=w449) -> ()  [unwired: 1 in, 2 out]
            n162 = call <vilib>:"Add State(s) to Queue__JKI_lib_State_Machine.vi"("State(s) in (\"\")"=w457, "State(s) at Back (\"\")"="Data: Redraw Scripts from UI" ("State(s) at Back (\"\")")) -> ("States Out"=w456:string)  [unwired: 13 in]
          }
          frame "Action: Replace Line" {
            n163 = Decimal String To Number(string=w470) -> (number=w467:i32)  [unwired: 2 in, 1 out]
            n164 = control-ref of="Script List"() -> (w469:refnum<vi>)
            n165 = call "Concatenate Submodule Name.vi"("name"="CmdEditor", "CSM Name"=w461) -> ("submodule name"=w459:string)  [unwired: 9 in]
            n166 = property class="LstBox (strict)"(reference=w469) -> (reference out=w465:refnum<vi>, "Item Names"=w468:string[])  [unwired: 1 in, 1 out]
            n167 = call "CSM - Send Message and Wait for Reply.vi"("Current Module(\"\" to generate a ID)"=w461, "Target Module"=w459, "State"="API: Get Command") -> ("Response"=w462:string)  [unwired: 6 in, 2 out]
            n168 = call "CSM - Revert Arguments-Safe String.vi"("Safe Argurment String"=w462) -> ("Origin Argurment String"=w463:string)  [unwired: 8 in]
            n169 = Replace Array Subset(array=w468, new element=w463, index=w467) -> (w466:string[])
            n170 = property class="LstBox (strict)"(reference=w465, "Item Names"=w466) -> ()  [unwired: 1 in, 2 out]
            n171 = call <vilib>:"Add State(s) to Queue__JKI_lib_State_Machine.vi"("State(s) in (\"\")"=w475, "State(s) at Back (\"\")"="Data: Redraw Scripts from UI" ("State(s) at Back (\"\")")) -> ("States Out"=w474:string)  [unwired: 13 in]
          }
          frame "Action: Delete Line" {
            n172 = Decimal String To Number(string=w482) -> (number=w476:i32)  [unwired: 2 in, 1 out]
            n173 = control-ref of="Script List"() -> (w481:refnum<vi>)
            n174 = property class="LstBox (strict)"(reference=w481) -> (reference out=w478:refnum<vi>, "Item Names"=w480:string[])  [unwired: 1 in, 1 out]
            n175 = Delete From Array(array=w480, index=w476) -> (array with subset deleted=w479:string[])  [unwired: 1 in, 1 out]
            n176 = property class="LstBox (strict)"(reference=w478, "Item Names"=w479) -> ()  [unwired: 1 in, 2 out]
            n177 = call <vilib>:"Add State(s) to Queue__JKI_lib_State_Machine.vi"("State(s) in (\"\")"=w487, "State(s) at Back (\"\")"="Data: Redraw Scripts from UI" ("State(s) at Back (\"\")")) -> ("States Out"=w486:string)  [unwired: 13 in]
          }
        }
      }
      n178 = Unbundle By Name(w10) -> ("Script"=w9:string)
    }
    frame Error {
    }
  }
  "Error out" <- w4
  "Script out" <- w2
